vi "RC_STM_Server.vi"() -> ()   [LabVIEW 2019, in "RemoteControl.STM.lvclass"]
uses:
  RemoteControl.STM.lvclass
  <vilib>/NI/STM/SubVIs/MetaDataElement.ctl
  <vilib>/NI/STM/Connection Manager/TCP/TCP Connection Method.ctl
  RemoteControl.STM.lvclass/RemoteControl.STM.ctl
  <vilib>/NI/STM/TCP/Write Meta Data (TCP Ref).vi
  <vilib>/NI/STM/TCP/Write Meta Data (TCP Clst).vi
  <vilib>/NI/STM/NI STM.lvlib
panel:
  in  "service name":string
  out "remote address":string
  out "command received":T1
  in  "Enum":T2(ring)
  out "data received":variant
  in  "stop":bool
  out "error out":errorcluster
  # "SERVER  (INSTRUMENT)"
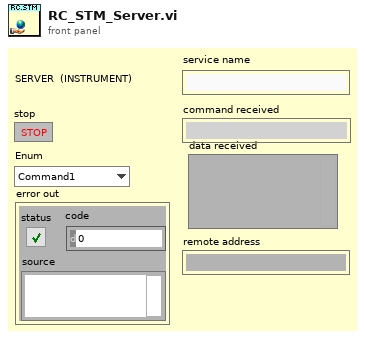
[diagram p1: front panel]
types:
  T1 = typedef "NI STM.lvlib/MetaDataElement.ctl" = string
  T2 = enum16{"Command1", "Command2", "Command3", "Command4", "HELP", "ACK", "CLOSE"}
  T3 = typedef "NI STM.lvlib/TCP Connection Method.ctl" = enum16{"Initialize", "Add Connection", "Set Properties", "Get Connection(s)", "Remove Connection", "Remove All Connections", "Get Connection Count"}
  T4 = typedef "NI STM.lvlib/TCP Connection Info.ctl" = cluster{"connection ID":refnum<k5>, "meta data":T1[]}
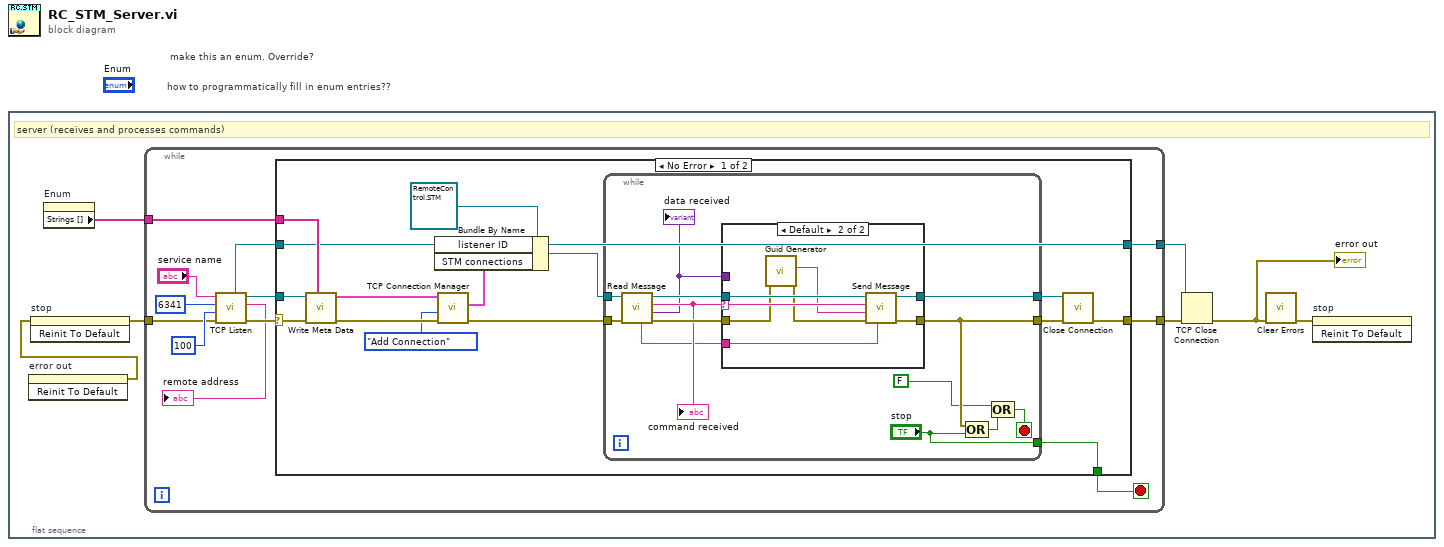
[diagram p0: block diagram]
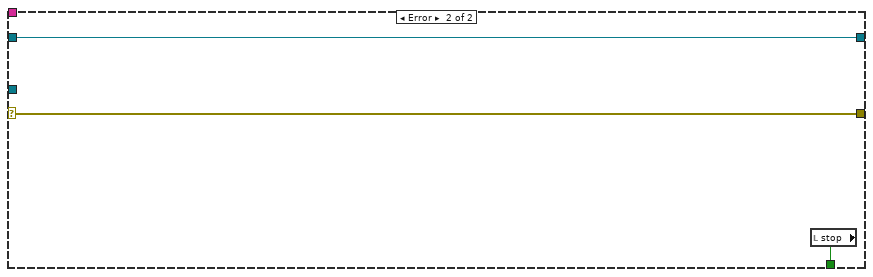
[diagram p3: hidden frame]
diagram:
  # "how to programmatically fill in enum entries??"
  # "make this an enum. Override?"
  n1 = flat-sequence {
    frame #0 {
      # "server (receives and processes commands)"
      n2 = invoke on="error out" class="Clust (strict)" method="Reinit To Default"() -> (error out=w4:errorcluster)  [unwired: 3 in, 2 out]
      n3 = invoke on="stop" class="Bool (strict)" method="Reinit To Default"(error in=w4) -> (error out=w7:errorcluster)  [unwired: 2 in, 2 out]
      n4 = property on="Enum" class="Enum (strict)"() -> ("Strings []"=w5:string[])  [unwired: 2 in, 2 out]
      n5 = while {
        tunnel: w7 -> [w14]
        tunnel: w5 -> [w13]
        tunnel: [w9] -> w3
        tunnel: [w8] -> w1
        stop <- w17 stop-if-true
        n6 = call <vilib>:"TCP Listen.vi"("error in (no error)"=w14, "timeout ms (wait forever: -1)"=100, "port"=u16 6341 ("remote port or service name"), "service name"="service name") -> ("error out"=w15:errorcluster, "remote address"=→"remote address":string, "connection ID"=w18:refnum<k5>, "listener ID"=w10:refnum<k5>)  [unwired: 3 in, 1 out]
        n7 = case shown="No Error" w15 {
          selector: w15 -> [w28 w58]
          tunnel: w18 -> [w23 _]
          tunnel: [w20 w60] -> w17
          tunnel: w13 -> [w29 _]
          tunnel: w10 -> [w21 w59]
          tunnel: [w22 w58] -> w9
          tunnel: [w21 w59] -> w8
          frame No Error {
            n8 = call-poly <vilib>:"Write Meta Data.vi"("meta data"=w29, "error in"=w28, "connection ID"=w23) -> ("error out"=w31:errorcluster, "connection info out"=w32:T4)  [unwired: 7 in]
            n9 = call <vilib>:"TCP Connection Manager.vi"("error in"=w31, "method"=TCP_Connection_Method."Add Connection", "connection in"=w32) -> ("error out"=w24:errorcluster, "all connections"=w26:T4[])  [unwired: 3 in, 4 out]
            n10 = Bundle By Name(cluster=refnum<class "RemoteControl.STM.lvclass"> refnum ("RemoteControl.STM in"), "listener ID"=w21, "STM connections"=w26) -> (w25:refnum<class "RemoteControl.STM.lvclass">)
            n11 = while {
              tunnel: [w46] -> w33
              tunnel: [w47] -> w34
              tunnel: ["stop"] -> w20
              tunnel: w24 -> [w42]
              tunnel: w25 -> [w41]
              stop <- w44 stop-if-true
              n12 = call-dynamic "Read Message.vi"("error in (no error)"=w42, "RemoteControl.STM in"=w41) -> ("error out"=w40:errorcluster, "Data"=w36:variant, "Command"=w39:string, "RemoteControl.STM out"=w38:refnum<class "RemoteControl.STM.lvclass">, "ID"=w37:string)  [unwired: 5 in]
              "data received" <- w36
              "command received" <- w39
              n13 = case shown="Default" w39 {
                selector: w39 -> [_ w54]
                tunnel: w38 -> [w48 w55]
                tunnel: [w48 w56] -> w47
                tunnel: w40 -> [w49 w51]
                tunnel: [w49 w57] -> w46
                tunnel: w36 -> [_ _]
                tunnel: w37 -> [_ w53]
                frame "" {
                }
                frame Default {
                  n14 = call <vilib>:"Guid Generator.vi"("error in (no error)"=w51) -> ("error out"=w50:errorcluster, "GUID"=w52:string)  [unwired: 9 in]
                  n15 = call-dynamic "Send Message.vi"("ID"=w53, "error in (no error)"=w50, "Data"=w52, "Command"=w54, "RemoteControl.STM in"=w55) -> ("error out"=w57:errorcluster, "RemoteControl.STM out"=w56:refnum<class "RemoteControl.STM.lvclass">)  [unwired: 5 in]
                }
              }
              n16 = Compound Arithmetic op=OR(w46, "stop") -> (w45:bool)
              n17 = Compound Arithmetic op=OR(FALSE ("value"), w45) -> (w44:bool)
            }
            n18 = call-dynamic "Close Connection.vi"("error in (no error)"=w33, "RemoteControl.STM in"=w34) -> ("error out"=w22:errorcluster)  [unwired: 8 in, 1 out]
          }
          frame Error {
            n19 = local read "stop"() -> (w60:bool)
          }
        }
      }
      n20 = TCP Close Connection(connection ID=w1, error in (no error)=w3) -> (error out=w2:errorcluster)  [unwired: 1 in, 1 out]
      "error out" <- w2
      n21 = call <vilib>:"Clear Errors.vi"("error in (no error)"=w2) -> ("error out"=w6:errorcluster)  [unwired: 5 in, 1 out]
      n22 = invoke on="stop" class="Bool (strict)" method="Reinit To Default"(error in=w6) -> ()  [unwired: 2 in, 3 out]
    }
  }
